vi "Set Cell ToolTipText.vi"(6 "ToolTipText":string, 8 "error in":errorcluster, 9 "Column":i32, 10 "Row":i32, 11 "SourceGrid in":refnum<class "SourceGrid.lvclass">) -> (0 "error out":errorcluster, 3 "SourceGrid out":refnum<class "SourceGrid.lvclass">)   [LabVIEW 2023, in "SourceGrid.lvlib" / "SourceGrid.lvclass"]
uses:
  SourceGrid.lvclass
  SourceGrid.lvclass/SourceGrid.ctl
  D:/git/Sourcegrid-LabVIEW/dll/SourceGrid.dll
  dll/SourceGrid.dll
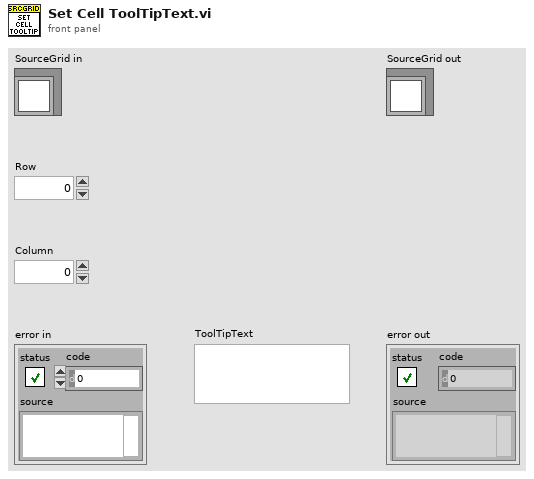
[diagram p1: front panel]
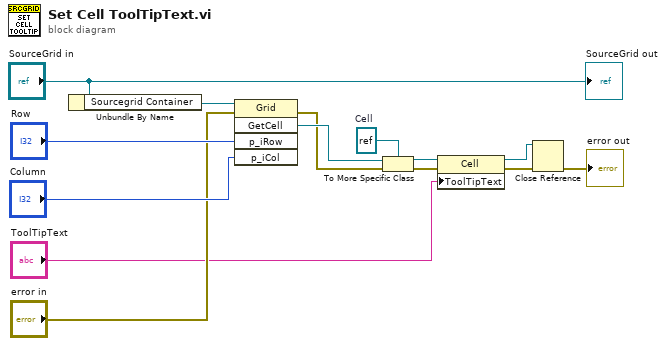
[diagram p0: block diagram]
diagram:
  w10 = refnum<k24> refnum  # Cell
  n1 = Unbundle By Name("SourceGrid in") -> ("Sourcegrid Container"=w13:refnum<k24>)
  n2 = invoke class="Grid" method="GetCell"(reference=w13, error in="error in", "p_iRow"="Row", "p_iCol"="Column") -> (error out=w8:errorcluster, "GetCell"=w9:refnum<k24>)  [unwired: 1 in, 3 out]
  n3 = To More Specific Class(target class=w10, reference=w9, error in=w8) -> (specific class reference=w5:refnum<k24>, error out=w6:errorcluster)
  n4 = property class="Cell"(reference=w5, error in=w6, "ToolTipText"="ToolTipText") -> (reference out=w1:refnum<k24>, error out=w3:errorcluster)
  n5 = Close Reference(reference=w1, error in (no error)=w3) -> (error out=→"error out":errorcluster)
  "SourceGrid out" <- "SourceGrid in"
